vi "Actor Core.vi"(8 "error in":errorcluster, 11 "Cli in":refnum<class "Cli.lvclass">) -> (0 "error out":errorcluster, 3 "Actor out":refnum<class "Actor.lvclass">)   [LabVIEW 2022 SP3, in "Cli.lvlib" / "Cli.lvclass"]
doc: "(<B>Filename</B>: Actor Framework.lvlib:Actor.lvclass:Actor Core.vi)\n\nReceives messages to the actor, reacts to them, and initiates any error handling that may shut the actor down.\n\nDescendant classes may override this VI to append parallel tasks for the actor to complete while it handles messages. Overrides use the Call Parent Class Method node."
uses:
  Cli.lvclass
  C:/Program Files (x86)/National Instruments/LabVIEW 2022/vi.lib/ActorFramework/Actor/Actor.lvclass
  <vilib>/ActorFramework/Actor/Actor.lvclass
  Tcp/Tcp/Tcp.lvclass
  Cli.lvclass/Cli.ctl
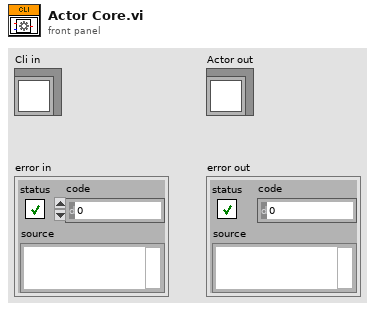
[diagram p1: front panel]
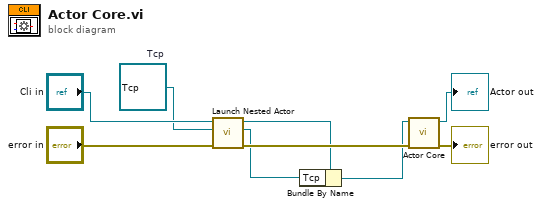
[diagram p0: block diagram]
diagram:
  w1 = refnum<class "Tcp.lvclass"> refnum  # Tcp
  n1 = call <vilib>:"Launch Nested Actor.vi"("error in (no error)"="error in", "Nested Actor"=w1, "Caller Actor in"="Cli in") -> ("error out"=w6:errorcluster, "Nested Actor's Enqueuer"=w3:refnum<class "Message Enqueuer.lvclass">, "Caller Actor out"=w4:refnum<class "Cli.lvclass">)  [unwired: 6 in]
  n2 = Bundle By Name(cluster=w4, "Tcp"=w3) -> (w2:refnum<class "Cli.lvclass">)
  n3 = call-parent "Actor Core.vi"("error in"=w6, "Actor in"=w2) -> ("error out"=→"error out":errorcluster, "Actor out"=→"Actor out":refnum<class "Actor.lvclass">)  [unwired: 8 in]
